vi "Get Reply Data.vi"(8 "error in (no error)":errorcluster, 9 "Data Msg in":refnum<class "Data Msg.lvclass">, 10 "Actor in":refnum<class "Actor.lvclass">, 11 "Replay Message":refnum<class "Read Data Msg.lvclass">) -> (0 "error out":errorcluster, 1 "Data Msg out":refnum<class "Data Msg.lvclass">, 2 "Actor out":refnum<class "Actor.lvclass">, 3 "Replay Message out":refnum<class "Read Data Msg.lvclass">, 4 "error?":bool)   [LabVIEW 2014, in "Observable Actor.lvlib" / "Read Data Msg.lvclass"]
doc: "(<B>Filename</B>: Actor Framework.lvlib:Message.lvclass:Do.vi)\n\nDefines what a message does when it is received by an actor. Generally, a message instructs an actor to invoke one of its methods. By default, this method does nothing. A child class must override it to define behavior. Create a child class by using the Actor Framework Message Maker dialog box."
uses:
  Read Data Msg.lvclass
  <vilib>/ActorFramework/Actor/Actor.lvclass
  Model/Data Msg/Data Msg.lvclass
  Extractor/AbstractExtractor/AbstractExtractor.lvclass
  Observable Actor.lvclass
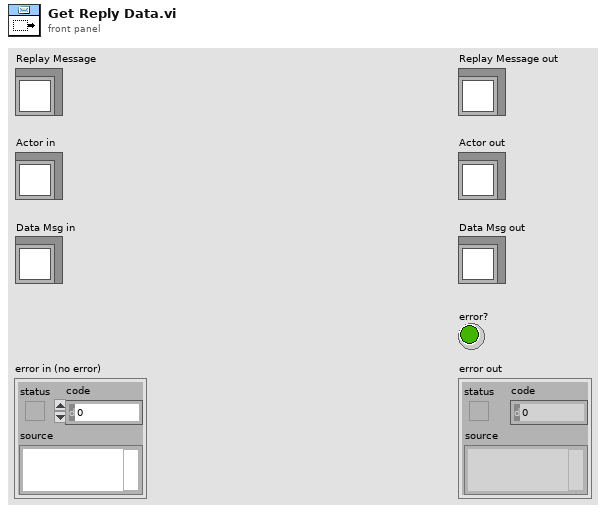
[diagram p1: front panel]
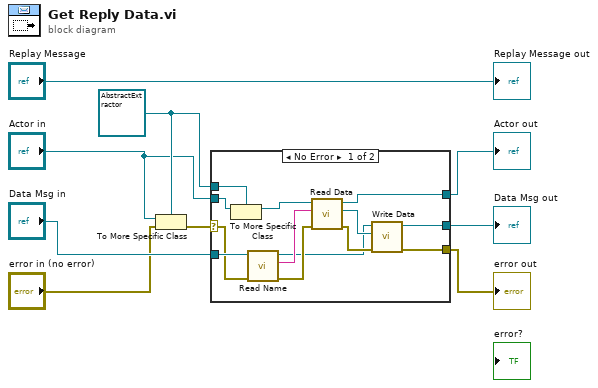
[diagram p0: block diagram]
diagram:
  w8 = refnum<class "AbstractExtractor.lvclass"> refnum ("Actor in")
  n1 = To More Specific Class(target class=w8, reference="Actor in", error in="error in (no error)") -> (error out=w9:errorcluster)  [unwired: 1 out]
  n2 = case shown="No Error" w9 {
    selector: w9 -> [w13 w25]
    tunnel: [w17 w25] -> w4
    tunnel: [w18 w24] -> w5
    tunnel: "Actor in" -> [w22 w24]
    tunnel: w8 -> [w21 _]
    tunnel: "Data Msg in" -> [w14 w23]
    tunnel: [w15 w23] -> w3
    frame No Error {
      n3 = To More Specific Class(target class=w21, reference=w22) -> (specific class reference=w20:refnum<class "AbstractExtractor.lvclass">)  [unwired: 1 in, 1 out]
      n4 = call-dynamic "Read Name.vi"("error in (no error)"=w13, "Data Msg in"=w14) -> ("error out"=w12:errorcluster, "Name"=w11:string, "Data Msg out"=w10:refnum<class "Data Msg.lvclass">)  [unwired: 7 in]
      n5 = call "Read Data.vi"("error in (no error)"=w12, "Name"=w11, "Observable Actor in"=w20) -> ("error out"=w16:errorcluster, "Data"=w19:refnum<class "AbstractData.lvclass">, "Observable Actor out"=w18:refnum<class "AbstractExtractor.lvclass">)  [unwired: 5 in, 1 out]
      n6 = call-dynamic "Write Data.vi"("error in (no error)"=w16, "AbstractData.lvclass"=w19, "Data Msg in"=w10) -> ("error out"=w17:errorcluster, "Data Msg out"=w15:refnum<class "Data Msg.lvclass">)  [unwired: 7 in]
    }
    frame Error {
    }
  }
  "error out" <- w4
  "Actor out" <- w5
  "Data Msg out" <- w3
  "Replay Message out" <- "Replay Message"
